vi "Set High Limit.vi"(8 "error in":errorcluster, 10 "High Limit":string, 11 "Object Entry in":refnum<class "Object Entry.lvclass">) -> (0 "error out":errorcluster, 3 "Object Entry out":refnum<class "Object Entry.lvclass">)   [LabVIEW 2020, in "CANopen.lvlib" / "Object Entry.lvclass"]
uses:
  Object Entry.lvclass
  Object Entry.lvclass/Object Entry.ctl
  Sub Object/Sub Object.lvclass
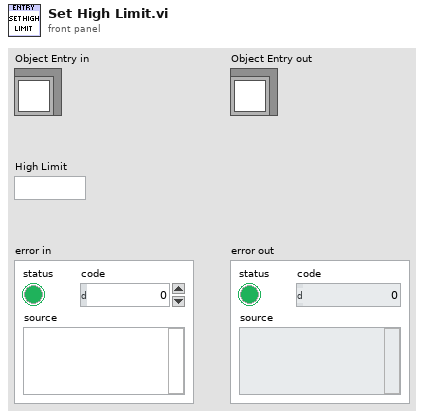
[diagram p1: front panel]
types:
  T1 = typedef "CANopen.lvlib/Object Type.ctl" = u8
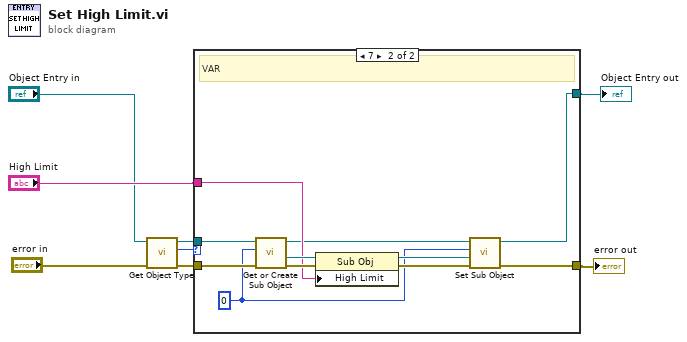
[diagram p0: block diagram]
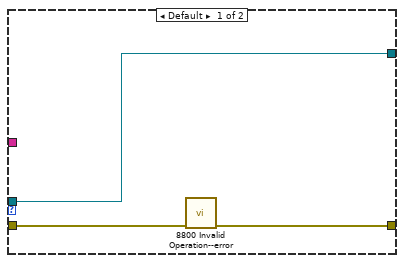
[diagram p2: hidden frame]
diagram:
  n1 = call "Get Object Type.vi"("error in"="error in", "Object Entry in"="Object Entry in") -> ("error out"=w6:errorcluster, "Object Type"=w7:T1, "Object Entry out"=w8:refnum<class "Object Entry.lvclass">)  [unwired: 7 in]
  n2 = case shown="7" w7 {
    tunnel: [w9 w14] -> w2
    tunnel: "High Limit" -> [_ w17]
    tunnel: w8 -> [w9 w20]
    tunnel: w6 -> [w11 w22]
    tunnel: [w10 w16] -> w1
    frame Default {
      n3 = call "8800 Invalid Operation--error.vi"("error in"=w11) -> ("error out"=w10:errorcluster)  [unwired: 9 in, 1 out]
    }
    frame 7 {
      w12 = u8 0 ("Sub Index")
      # "VAR"
      n4 = call "Get or Create Sub Object.vi"("error in"=w22, "Sub Index"=w12, "Obj Entry in"=w20) -> ("error out"=w21:errorcluster, "Sub Object"=w18:refnum<class "Sub Object.lvclass">, "Obj Entry out"=w15:refnum<class "Object Entry.lvclass">)  [unwired: 6 in]
      n5 = property class="Sub Obj"(reference=w18, error in=w21, "High Limit"=w17) -> (reference out=w13:refnum<class "Sub Object.lvclass">, error out=w19:errorcluster)
      n6 = call "Set Sub Object.vi"("error in"=w19, "Sub Object"=w13, "Sub Index"=w12, "Obj Entry in"=w15) -> ("error out"=w16:errorcluster, "Obj Entry out"=w14:refnum<class "Object Entry.lvclass">)  [unwired: 6 in]
    }
  }
  "error out" <- w1
  "Object Entry out" <- w2
